vi "SR760 get data.VI"(8 "error in 2":errorcluster, 10 "active trace":i8 min=0 max=1, 11 "GPIB address":string="10") -> (0 "error out":T1, 3 "trace":dbl[](graph))   [LabVIEW 2023]
doc: "This subVI implements the binary data transfer function (SPEB) of the SR760/SR770 and demonstrates how the actual Y values are obtained from the data downloaded from the SR760/770 .\nACTIVE TRACE determines which trace will be displayed in graph TRACE .\nX and 'Y=' display the current marker X & Y positions respectively and UNITS displays the units of the Y reading ."
panel:
  in  "type indicator":i16[](array[numeric])
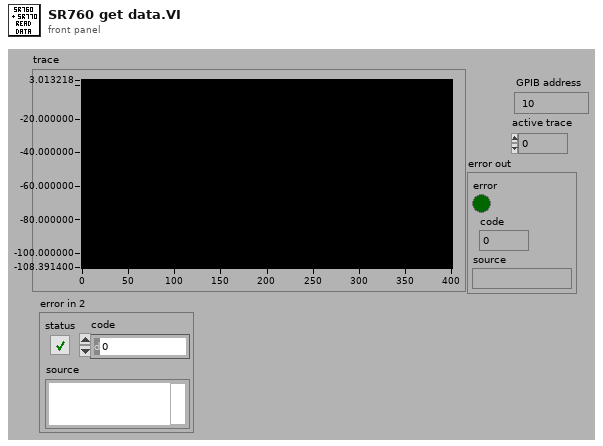
[diagram p1: front panel]
types:
  T1 = cluster{"error":bool, "code":i32, "source":string}
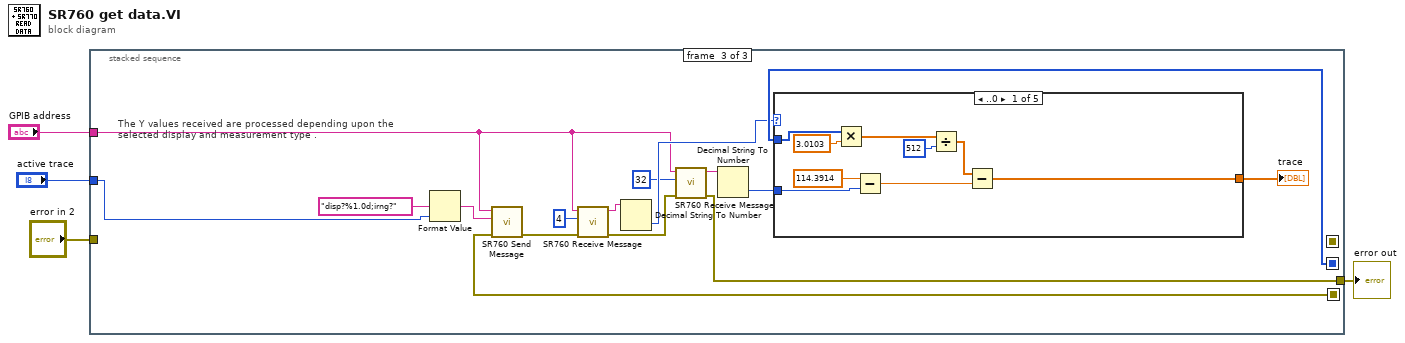
[diagram p0: block diagram]
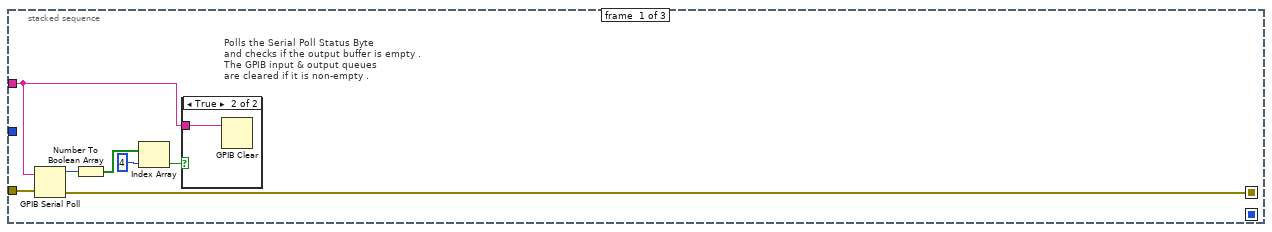
[diagram p2: hidden frame]
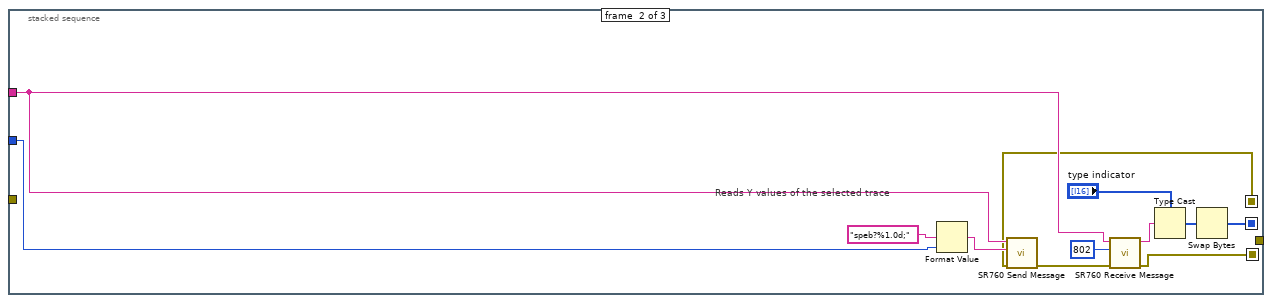
[diagram p4: hidden frame]
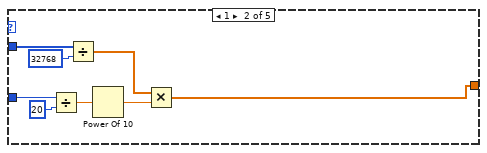
[diagram p5: hidden frame]
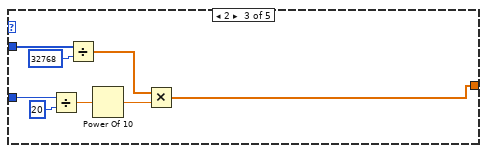
[diagram p6: hidden frame]
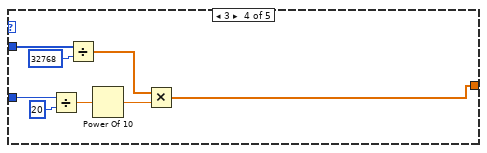
[diagram p7: hidden frame]
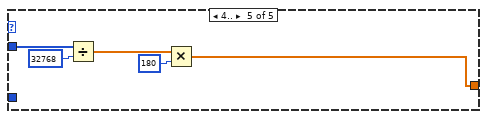
[diagram p8: hidden frame]
diagram:
  n1 = stacked-sequence {
    seq-local: [_ w19 _] -> [_ _ w40]
    seq-local: [w5 _ _] -> [_ w14 _]
    seq-local: [_ w13 _] -> [_ _ w26]
    tunnel: "GPIB address" -> [w7 w24 w29]
    tunnel: "active trace" -> [_ w18 w37]
    tunnel: "error in 2" -> [w6 _ _]
    tunnel: [_ _ w25] -> w1
    frame #0 {
      # "Polls the Serial Poll Status Byte\nand checks if the output buffer is empty .\nThe GPIB input & output queues \nare cleared if it is non-empty ."
      n2 = GPIB Serial Poll(0:w7, 1:w6) -> (2:w11:i16, 4:w5:errorcluster)  [unwired: 1 out]
      n3 = Number To Boolean Array(number=w11) -> (Boolean array=w10:bool[])
      n4 = Index Array(array=w10, index=4) -> (element=w8:bool)
      n5 = case shown="True" w8 {
        tunnel: w7 -> [_ w12]
        frame False {
        }
        frame True {
          n6 = GPIB Clear(3:w12) -> ()  [unwired: 1 in, 2 out]
        }
      }
    }
    frame #1 {
      # "Reads Y values of the selected trace"
      n7 = Format Value(format string="speb?%1.0d;", value (0)=w18) -> (output string=w16:string)  [unwired: 1 in]
      n8 = call <instrlib>:"SR760 Send Message.vi"("address string"=w24, "write buffer"=w16, "error in"=w14) -> ("error out"=w23:T1)  [unwired: 4 in, 2 out]
      n9 = call <instrlib>:"SR760 Receive Message.vi"("address string"=w24, "byte count"=802, "error in"=w23) -> ("read buffer"=w22:string, "error out"=w13:T1)  [unwired: 4 in, 1 out]
      n10 = Type Cast(type="type indicator", x=w22) -> (*(type *) &x=w20:i16[])
      n11 = Swap Bytes(anything=w20) -> (byte swapped=w19:i16[])
    }
    frame #2 {
      # "The Y values received are processed depending upon the \nselected display and measurement type ."
      n12 = Format Value(format string="disp?%1.0d;irng?", value (0)=w37) -> (output string=w36:string)  [unwired: 1 in]
      n13 = call <instrlib>:"SR760 Send Message.vi"("address string"=w29, "write buffer"=w36, "error in"=w26) -> ("error out"=w34:T1)  [unwired: 4 in, 2 out]
      n14 = call <instrlib>:"SR760 Receive Message.vi"("address string"=w29, "byte count"=4, "error in"=w34) -> ("read buffer"=w33:string, "error out"=w31:T1)  [unwired: 4 in, 1 out]
      n15 = Decimal String To Number(string=w33) -> (number=w32:i32)  [unwired: 2 in, 1 out]
      n16 = call <instrlib>:"SR760 Receive Message.vi"("address string"=w29, "byte count"=32, "error in"=w31) -> ("read buffer"=w28:string, "error out"=w25:T1)  [unwired: 4 in, 1 out]
      n17 = Decimal String To Number(string=w28) -> (number=w27:i32)  [unwired: 2 in, 1 out]
      n18 = case shown="..0" w32 {
        tunnel: w40 -> [w43 w56 w64 w72 w77]
        tunnel: [w41 w51 w59 w67 w75] -> w39
        tunnel: w27 -> [w42 w50 w58 w66 _]
        frame ..0 {
          n19 = Multiply(x=w43, y=3.0103) -> (x*y=w47:dbl[])
          n20 = Subtract(x=114.3914, y=w42) -> (x-y=w44:dbl)
          n21 = Divide(x=w47, y=512) -> (x/y=w48:dbl[])
          n22 = Subtract(x=w48, y=w44) -> (x-y=w41:dbl[])
        }
        frame 1 {
          n23 = Divide(x=w50, y=20) -> (x/y=w53:dbl)
          n24 = Divide(x=w56, y=32768) -> (x/y=w54:dbl[])
          n25 = Power Of 10(x=w53) -> (10^x=w52:dbl)
          n26 = Multiply(x=w54, y=w52) -> (x*y=w51:dbl[])
        }
        frame 2 {
          n27 = Divide(x=w58, y=20) -> (x/y=w61:dbl)
          n28 = Divide(x=w64, y=32768) -> (x/y=w62:dbl[])
          n29 = Power Of 10(x=w61) -> (10^x=w60:dbl)
          n30 = Multiply(x=w62, y=w60) -> (x*y=w59:dbl[])
        }
        frame 3 {
          n31 = Divide(x=w66, y=20) -> (x/y=w69:dbl)
          n32 = Divide(x=w72, y=32768) -> (x/y=w70:dbl[])
          n33 = Power Of 10(x=w69) -> (10^x=w68:dbl)
          n34 = Multiply(x=w70, y=w68) -> (x*y=w67:dbl[])
        }
        frame 4.. {
          n35 = Divide(x=w77, y=32768) -> (x/y=w76:dbl[])
          n36 = Multiply(x=w76, y=180) -> (x*y=w75:dbl[])
        }
      }
      "trace" <- w39
    }
  }
  "error out" <- w1
